vi "programControlQueueFGV.vi"(8 "error in (no error)":errorcluster, 10 "message in":T1, 11 "Enum":T2) -> (0 "error out":errorcluster, 2 "message out":T1)   [LabVIEW 2017, in "programControl.lvlib"]
uses:
  programControl.lvlib
  TypeDefs/queueFGVState.ctl
  TypeDefs/message.ctl
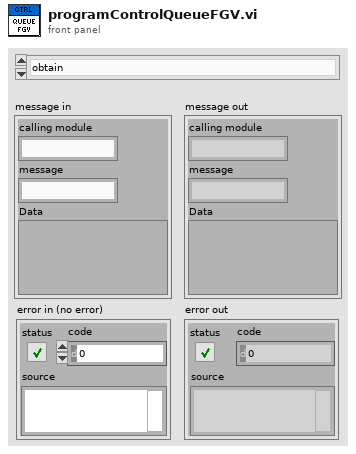
[diagram p1: front panel]
types:
  T1 = typedef "programControl.lvlib/message.ctl" = cluster{"calling module":string, "message":string, "Data":variant}
  T2 = typedef "programControl.lvlib/queueFGVState.ctl" = enum16{"obtain", "enqueue (low priority)", "enqueue (high priority)", "dequeue", "release"}
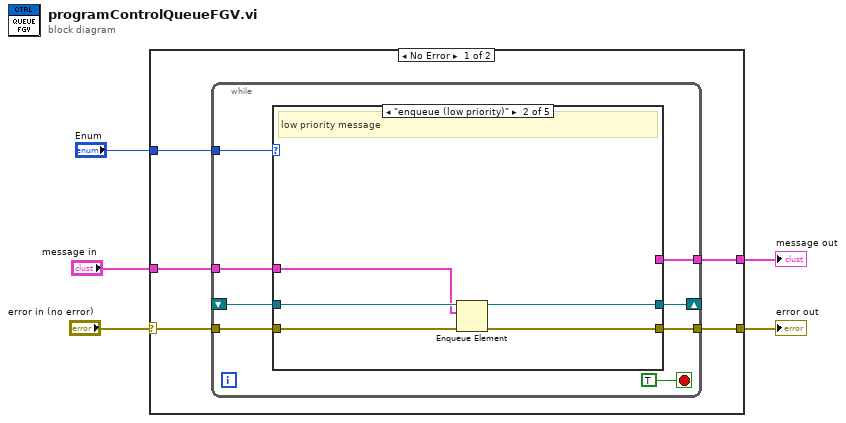
[diagram p0: block diagram]
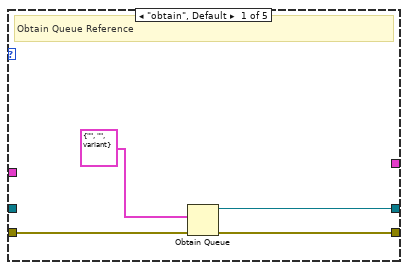
[diagram p2: hidden frame]
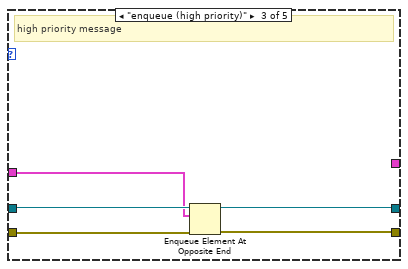
[diagram p3: hidden frame]
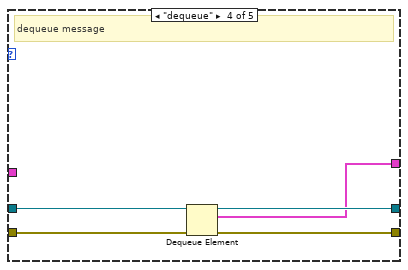
[diagram p4: hidden frame]
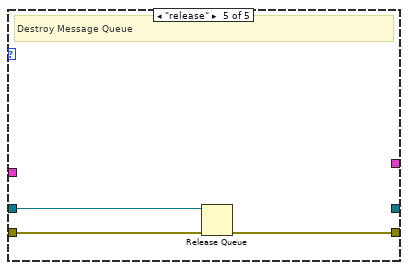
[diagram p5: hidden frame]
diagram:
  n1 = case shown="No Error" "error in (no error)" {
    selector: "error in (no error)" -> [w10 w41]
    tunnel: [w8 w41] -> w4
    tunnel: "Enum" -> [w9 _]
    tunnel: [w7 _] -> w2
    tunnel: "message in" -> [w6 _]
    frame No Error {
      n2 = while {
        tunnel: w10 -> [w16]
        tunnel: w9 -> [w17]
        tunnel: [w15] -> w8
        shift-right: [w14] -> _
        shift-left: _ -> [w13]
        tunnel: [w12] -> w7
        tunnel: w6 -> [w11]
        stop <- TRUE stop-if-true
        n3 = case shown="\"enqueue (low priority)\"" w17 {
          tunnel: w16 -> [w22 w27 w32 w37 w40]
          tunnel: [w21 w26 w31 w36 w39] -> w15
          tunnel: [w20 w25 w30 w35 _] -> w14
          tunnel: w13 -> [_ w24 w29 w34 w38]
          tunnel: [_ _ _ w33 _] -> w12
          tunnel: w11 -> [_ w23 w28 _ _]
          frame "obtain", Default {
            # "Obtain Queue Reference"
            n4 = Obtain Queue(element data type=T1 {"calling module"="", "message"="", "Data"=variant} ("message"), error in (no error)=w22) -> (queue out=w20:refnum<queue>, error out=w21:errorcluster)  [unwired: 3 in, 1 out]
          }
          frame "enqueue (low priority)" {
            # "low priority message"
            n5 = Enqueue Element(queue=w24, element=w23, error in (no error)=w27) -> (queue out=w25:refnum<queue>, error out=w26:errorcluster)  [unwired: 1 in, 1 out]
          }
          frame "enqueue (high priority)" {
            # "high priority message"
            n6 = Enqueue Element At Opposite End(queue=w29, element=w28, error in (no error)=w32) -> (queue out=w30:refnum<queue>, error out=w31:errorcluster)  [unwired: 1 in, 1 out]
          }
          frame "dequeue" {
            # "dequeue message"
            n7 = Dequeue Element(queue=w34, error in (no error)=w37) -> (queue out=w35:refnum<queue>, element=w33:T1, error out=w36:errorcluster)  [unwired: 1 in, 1 out]
          }
          frame "release" {
            # "Destroy Message Queue"
            n8 = Release Queue(queue=w38, error in (no error)=w40) -> (error out=w39:errorcluster)  [unwired: 1 in, 2 out]
          }
        }
      }
    }
    frame Error {
    }
  }
  "error out" <- w4
  "message out" <- w2
